vi "OnDiagnosticsMessage Event Callback.vi"(4 "Camera Diagnostics Message":refnum<vi>, 5 "Event Data":T1, 6 "Control Ref":refnum<k24>, 7 "Event Common Data":T2) -> ()   [LabVIEW 2015]
uses:
  C:/code/Host/Installer/Scientific Camera Interfaces/LabVIEW/64_bit/Library_X64/Thorlabs.TSI.TLCameraInterfaces.dll
  code/Host/Installer/Scientific Camera Interfaces/LabVIEW/64_bit/Library_X64/Thorlabs.TSI.TLCameraInterfaces.dll
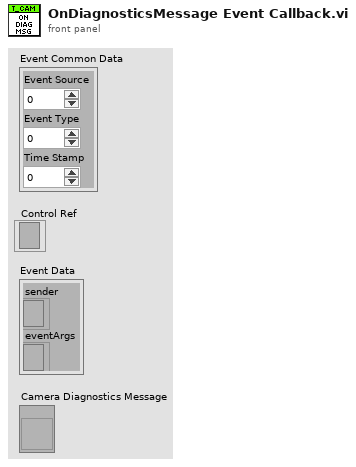
[diagram p1: front panel]
types:
  T1 = cluster{"sender":refnum<k24>, "eventArgs":refnum<k24>}
  T2 = cluster{"Event Source":i32, "Event Type":u32, "Time Stamp":u32}
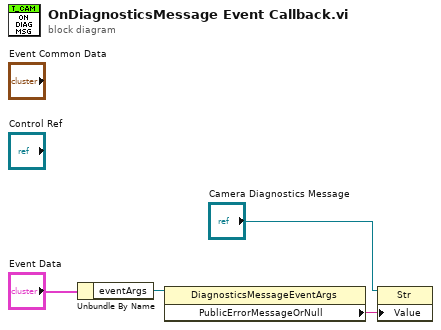
[diagram p0: block diagram]
diagram:
  n1 = Unbundle By Name("Event Data") -> ("eventArgs"=w4:refnum<k24>)
  n2 = property class="DiagnosticsMessageEventArgs"(reference=w4) -> ("PublicErrorMessageOrNull"=w3:string)  [unwired: 1 in, 2 out]
  n3 = property class="Str"(reference="Camera Diagnostics Message", "Value"=w3) -> ()  [unwired: 1 in, 2 out]
